vi "A_7.vi"() -> ()   [LabVIEW 2020]
panel:
  in  "stop":bool
  out "Elapsed time [ms]":u32
  in  "Reset Timer":bool
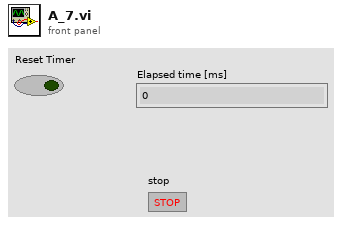
[diagram p1: front panel]
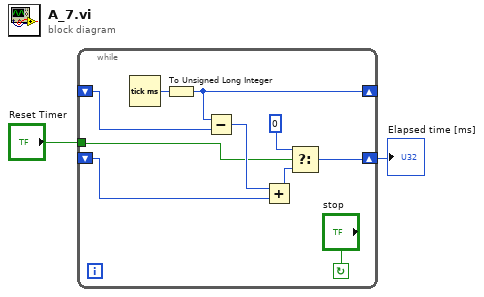
[diagram p0: block diagram]
diagram:
  n1 = while {
    shift-right: [w10] -> _
    shift-left: _ -> [w11]
    shift-right: [w4] -> w1
    shift-left: _ -> [w8]
    tunnel: "Reset Timer" -> [w6]
    stop <- "stop" continue-if-true
    n2 = Tick Count (ms)() -> (millisecond timer value=w12:u32)
    n3 = To Unsigned Long Integer(number=w12) -> (unsigned 32bit integer=w10:u32)
    n4 = Subtract(x=w10, y=w11) -> (x-y=w9:u32)
    n5 = Add(x=w9, y=w8) -> (x+y=w5:u32)
    n6 = Select(t=u32 0, s=w6, f=w5) -> (s? t:f=w4:u32)
  }
  "Elapsed time [ms]" <- w1
